vi "_시리얼_Mark10-설정 (이동속도).vi"(4 "속도(mm/min)":dbl, 5 "시리얼 포트":refnum<visa-resource-name>="COM5") -> (2 "VISA 리소스 이름 출력":refnum<visa-resource-name>)   [LabVIEW 2015]
panel:
  out "전송 문자열":string
  # "MARK10 이동속도 설정"
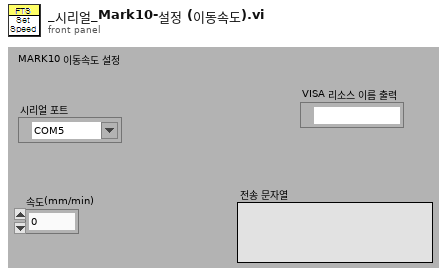
[diagram p1: front panel]
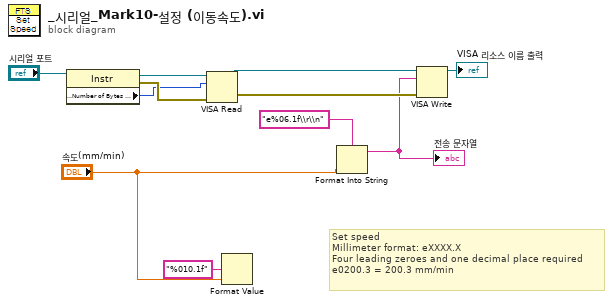
[diagram p0: block diagram]
diagram:
  # "Set speed\nMillimeter format: eXXXX.X\nFour leading zeroes and one decimal place required\ne0200.3 = 200.3 mm/min"
  n1 = property class="Instr"(reference="시리얼 포트") -> (reference out=w11:refnum<visa-resource-name>, error out=w9:errorcluster, "Serial Settings:Number of Bytes at Serial Port"=w6:u32)  [unwired: 1 in]
  n2 = VISA Read(VISA resource name=w11, byte count=w6, error in (no error)=w9) -> (VISA resource name out=w8:refnum<visa-resource-name>, error out=w7:errorcluster)  [unwired: 2 out]
  n3 = Format Value(format string="%010.1f" ("포맷 문자열"), value (0)="속도(mm/min)") -> ()  [unwired: 1 in, 1 out]
  n4 = Format Into String(format string="e%06.1f\\r\\n" ("포맷 문자열"), "속도(mm/min)") -> (resulting string=w4:string)  [unwired: 2 in, 1 out]
  "전송 문자열" <- w4
  n5 = VISA Write(VISA resource name=w8, write buffer=w4, error in (no error)=w7) -> (VISA resource name out=→"VISA 리소스 이름 출력":refnum<visa-resource-name>)  [unwired: 2 out]
